vi "ControlList.vi"() -> (0 "Tab Control":cluster{"Control Path":string, "Data":variant}[](array[cluster]), 1 "BigCluster":cluster{"Control Path":string, "Data":variant}[](array[cluster]), 2 "Cluster":cluster{"Control Path":string, "Data":variant}[](array[cluster]), 3 "Basic":cluster{"Control Path":string, "Data":variant}[](array[cluster]), 4 "SubPanel":cluster{"Control Path":string, "Data":variant}[](array[cluster]), 6 "BasicArray":cluster{"Control Path":string, "Data":variant}[](array[cluster]))   [LabVIEW 2016, in "Drona Test.lvlib"]
uses:
  Drona Test.lvlib
  TestHelper/controls/Level2.ctl
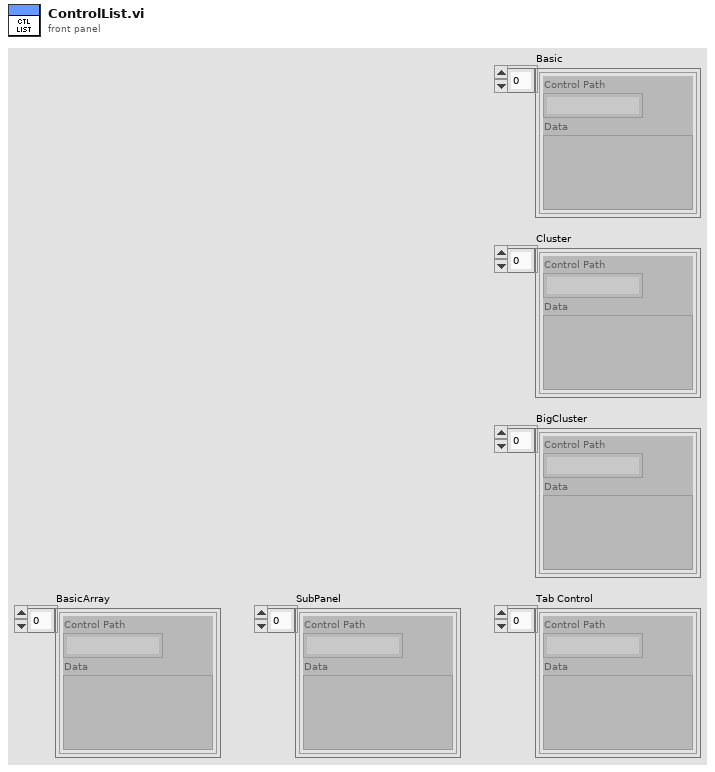
[diagram p1: front panel]
types:
  T1 = typedef "Level2.ctl" = cluster{"Numeric_cluster":dbl, "Boolean_cluster":bool, "target":string}
  T2 = cluster{"Control Path":string, "BigCluster":cluster{"Numeric_cluster":dbl, "Boolean_cluster":bool, "String_cluster":string, "Level1":cluster{"Numeric_cluster":dbl, "Boolean_cluster":bool, "String_cluster":string, "Level2":T1}}}
  T3 = cluster{"Control Path":string, "Data":cluster{"Numeric_cluster":dbl, "Boolean_cluster":bool, "String_cluster":string}}
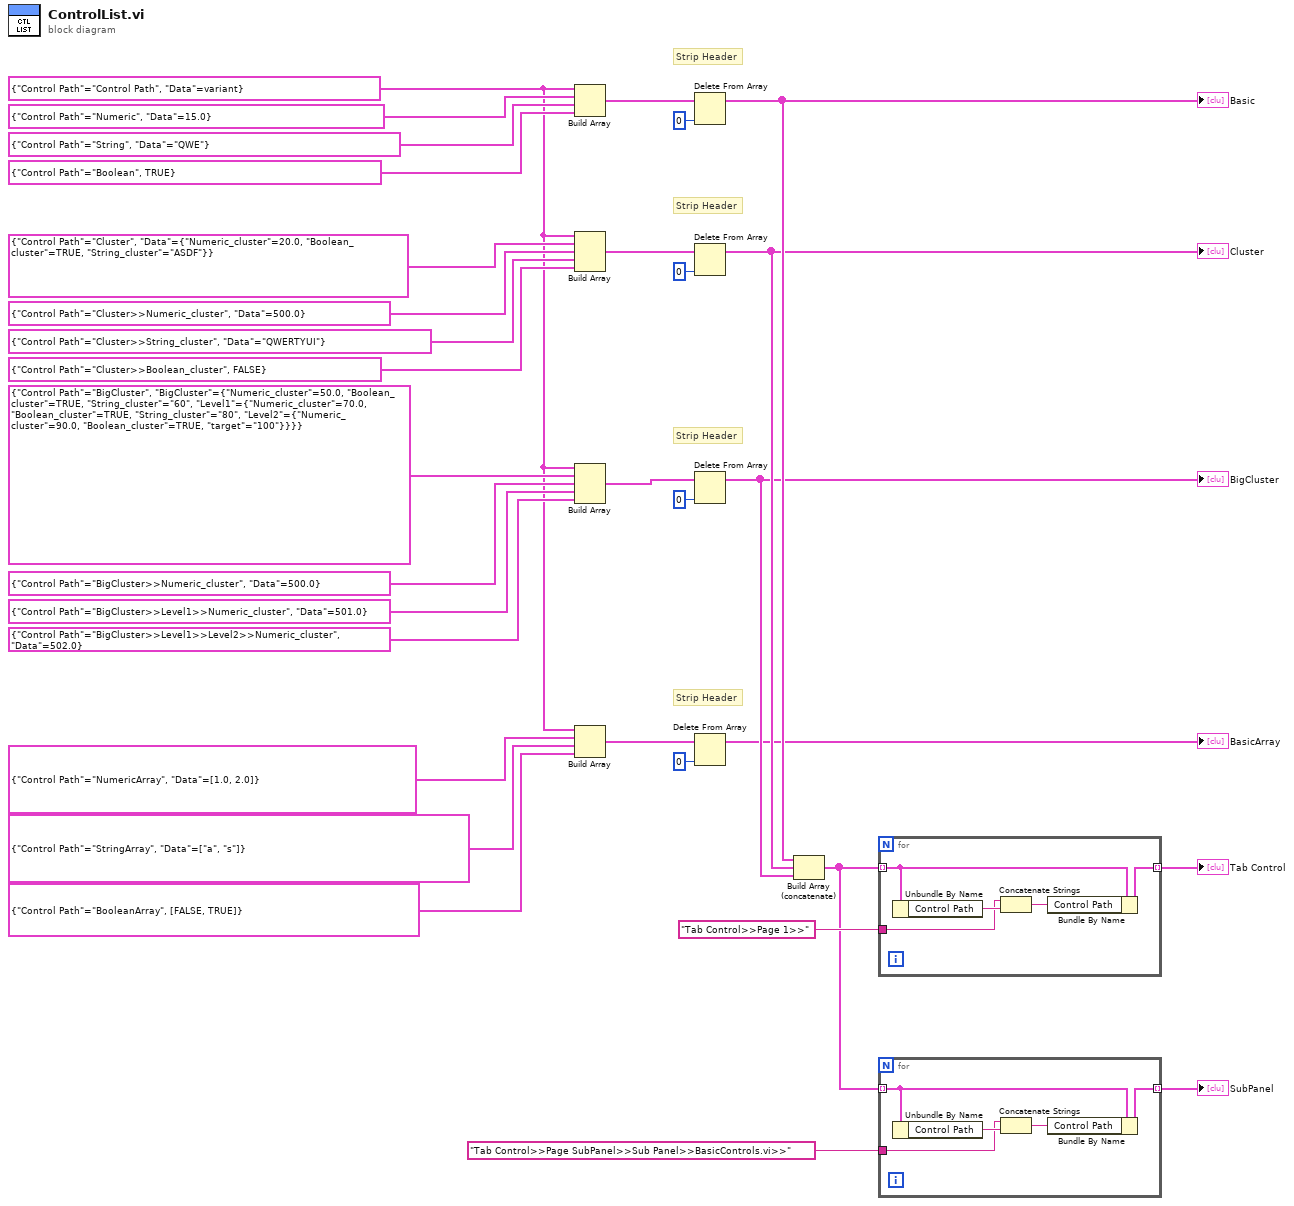
[diagram p0: block diagram]
diagram:
  w2 = cluster{"Control Path":string, "Data":variant} {"Control Path"="Control Path", "Data"=variant}
  # "Strip Header"
  # "Strip Header"
  # "Strip Header"
  # "Strip Header"
  n1 = Build Array(w2, cluster{"Control Path":string, "Data":dbl} {"Control Path"="Numeric", "Data"=15.0}, cluster{"Control Path":string, "Data":string} {"Control Path"="String", "Data"="QWE"}, cluster{"Control Path":string, bool} {"Control Path"="Boolean", TRUE}) -> (w28:cluster{"Control Path":string, "Data":variant}[])
  n2 = Build Array(w2, T3 {"Control Path"="Cluster", "Data"={"Numeric_cluster"=20.0, "Boolean_cluster"=TRUE, "String_cluster"="ASDF"}}, cluster{"Control Path":string, "Data":dbl} {"Control Path"="Cluster>>Numeric_cluster", "Data"=500.0}, cluster{"Control Path":string, "Data":string} {"Control Path"="Cluster>>String_cluster", "Data"="QWERTYUI"}, cluster{"Control Path":string, bool} {"Control Path"="Cluster>>Boolean_cluster", FALSE}) -> (w22:cluster{"Control Path":string, "Data":variant}[])
  n3 = Build Array(w2, T2 {"Control Path"="BigCluster", "BigCluster"={"Numeric_cluster"=50.0, "Boolean_cluster"=TRUE, "String_cluster"="60", "Level1"={"Numeric_cluster"=70.0, "Boolean_cluster"=TRUE, "String_cluster"="80", "Level2"={"Numeric_cluster"=90.0, "Boolean_cluster"=TRUE, "target"="100"}}}}, cluster{"Control Path":string, "Data":dbl} {"Control Path"="BigCluster>>Numeric_cluster", "Data"=500.0}, cluster{"Control Path":string, "Data":dbl} {"Control Path"="BigCluster>>Level1>>Numeric_cluster", "Data"=501.0}, cluster{"Control Path":string, "Data":dbl} {"Control Path"="BigCluster>>Level1>>Level2>>Numeric_cluster", "Data"=502.0}) -> (w21:cluster{"Control Path":string, "Data":variant}[])
  n4 = Build Array(w2, cluster{"Control Path":string, "Data":dbl[]} {"Control Path"="NumericArray", "Data"=[1.0, 2.0]}, cluster{"Control Path":string, "Data":string[]} {"Control Path"="StringArray", "Data"=["a", "s"]}, cluster{"Control Path":string, bool[]} {"Control Path"="BooleanArray", [FALSE, TRUE]}) -> (w7:cluster{"Control Path":string, "Data":variant}[])
  n5 = Delete From Array(array=w28, index=0) -> (array with subset deleted=w15:cluster{"Control Path":string, "Data":variant}[])  [unwired: 1 in, 1 out]
  "Basic" <- w15
  n6 = Delete From Array(array=w22, index=0) -> (array with subset deleted=w14:cluster{"Control Path":string, "Data":variant}[])  [unwired: 1 in, 1 out]
  "Cluster" <- w14
  n7 = Delete From Array(array=w21, index=0) -> (array with subset deleted=w13:cluster{"Control Path":string, "Data":variant}[])  [unwired: 1 in, 1 out]
  "BigCluster" <- w13
  n8 = Delete From Array(array=w7, index=0) -> (array with subset deleted=→"BasicArray":cluster{"Control Path":string, "Data":variant}[])  [unwired: 1 in, 1 out]
  n9 = Build Array (concatenate)(w15, w14, w13) -> (w8:cluster{"Control Path":string, "Data":variant}[])
  n10 = for {
    tunnel: w8 -> [w37] mode=indexing
    tunnel: [w36] -> w11 mode=indexing
    tunnel: "Tab Control>>Page 1>>" ("Control Path") -> [w34]
    n11 = Unbundle By Name(w37) -> ("Control Path"=w35:string)
    n12 = Concatenate Strings(w34, w35) -> (w33:string)
    n13 = Bundle By Name(cluster=w37, "Control Path"=w33) -> (w36:cluster{"Control Path":string, "Data":variant})
  }
  "Tab Control" <- w11
  n14 = for {
    tunnel: w8 -> [w42] mode=indexing
    tunnel: [w41] -> w10 mode=indexing
    tunnel: "Tab Control>>Page SubPanel>>Sub Panel>>BasicControls.vi>>" ("Control Path") -> [w39]
    n15 = Unbundle By Name(w42) -> ("Control Path"=w40:string)
    n16 = Concatenate Strings(w39, w40) -> (w38:string)
    n17 = Bundle By Name(cluster=w42, "Control Path"=w38) -> (w41:cluster{"Control Path":string, "Data":variant})
  }
  "SubPanel" <- w10
